vi "Calculate Odd Parity Bit.vi"(0 "Byte":u8 format="%02x", 11 "error in (no error)":errorcluster) -> (4 "Odd Parity Bit":u8, 15 "error out":errorcluster)   [LabVIEW 2018, in "MIPI RFFE API.lvlib"]
uses:
  MIPI RFFE API.lvlib
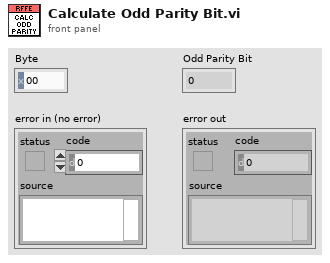
[diagram p1: front panel]
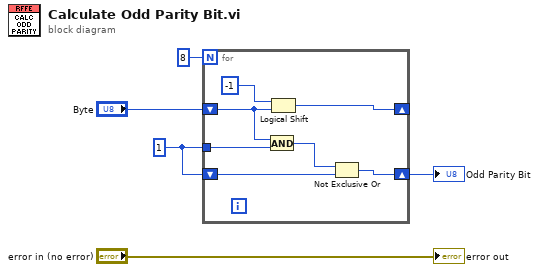
[diagram p0: block diagram]
diagram:
  w1 = u8 1
  n1 = for {
    N: 8 -> [_]
    shift-right: [w11] -> w3
    shift-left: w1 -> [w12]
    tunnel: w1 -> [w10]
    shift-right: [w6] -> _
    shift-left: "Byte" -> [w8]
    n2 = And(x=w8, y=w10) -> (x .and. y?=w9:u8)
    n3 = Logical Shift(y=i16 -1, x=w8) -> (x << y=w6:u8)
    n4 = Not Exclusive Or(1:w12, 2:w9) -> (0:w11:u8)
  }
  "Odd Parity Bit" <- w3
  "error out" <- "error in (no error)"
